vi "Get Write Map.vi"(1 "Setup":T2) -> (0 "Write Map OUT":T1)   [LabVIEW 2024, in "EtherCAT Model.lvlib"]
uses:
  EtherCAT Model.lvlib
  EtherCAT Configuration.ctl
  Write Context Typedef.ctl
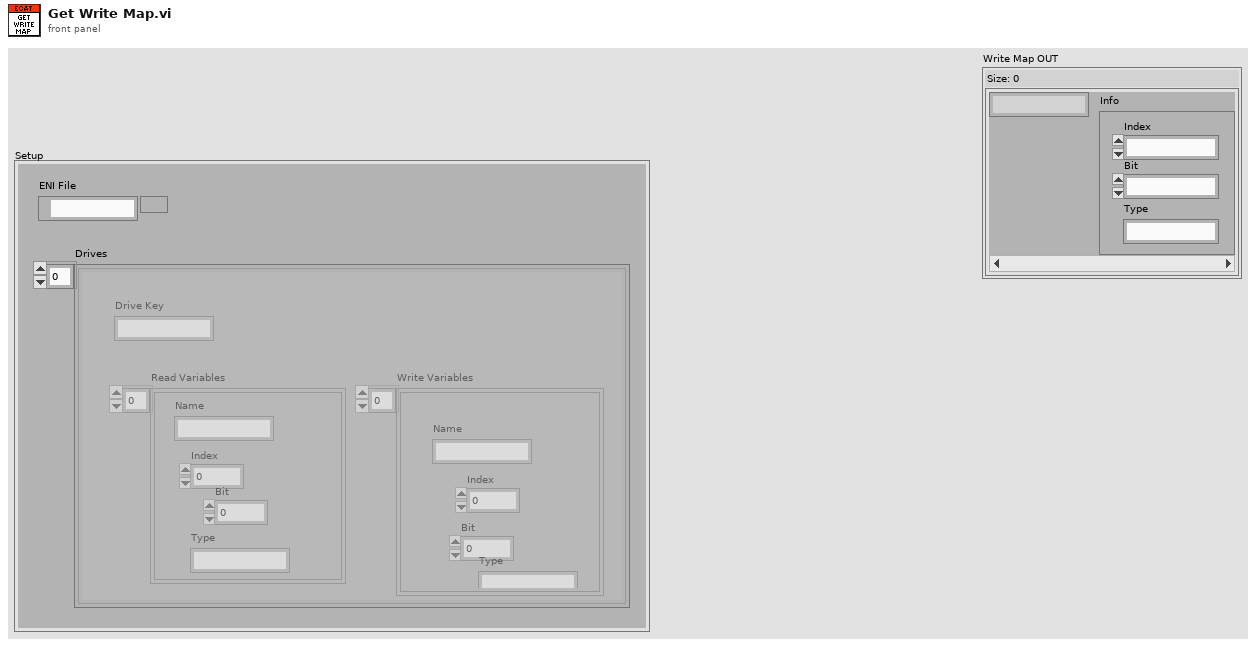
[diagram p1: front panel]
types:
  T1 = typedef "EtherCAT Model.lvlib/Write Context Typedef.ctl" = map{string, cluster{"Index":i32, "Bit":u8, "Type":string}}
  T2 = typedef "EtherCAT Configuration.ctl" = cluster{"ENI File":path, "Drives":cluster{"Drive Key":string, "Read Variables":cluster{"Name":string, "Index":i32, "Bit":u8, "Type":string}[], "Write Variables":cluster{"Name":string, "Index":i32, "Bit":u8, "Type":string}[]}[]}
  T3 = cluster{"Drive Key":string, "Read Variables":cluster{"Name":string, "Index":i32, "Bit":u8, "Type":string}[], "Write Variables":cluster{"Name":string, "Index":i32, "Bit":u8, "Type":string}[]}[]
  T4 = cluster{"Name":string, "Index":i32, "Bit":u8, "Type":string}[]
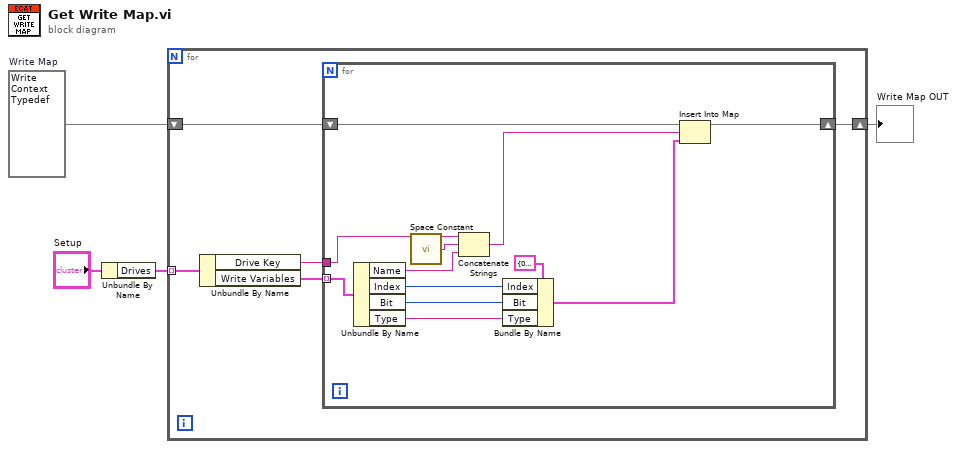
[diagram p0: block diagram]
diagram:
  w2 = T1 {}  # Write Map
  n1 = Unbundle By Name("Setup") -> ("Drives"=w3:T3)
  n2 = for {
    tunnel: w3 -> [w9] mode=indexing
    shift-right: [w5] -> w1
    shift-left: w2 -> [w6]
    n3 = Unbundle By Name(w9) -> ("Drive Key"=w7:string, "Write Variables"=w8:T4)
    n4 = for {
      tunnel: w8 -> [w21] mode=indexing
      tunnel: w7 -> [w20]
      shift-right: [w10] -> w5
      shift-left: w6 -> [w16]
      n5 = Unbundle By Name(w21) -> ("Name"=w18:string, "Index"=w14:i32, "Bit"=w13:u8, "Type"=w12:string)
      n6 = call <vilib>:"Space Constant.vi"() -> ("String"=w19:string)
      n7 = Concatenate Strings(w20, w19, w18) -> (w17:string)
      n8 = Bundle By Name(cluster=cluster{"Index":i32, "Bit":u8, "Type":string} {"Index"=0, "Bit"=0, "Type"=""} ("Info"), "Index"=w14, "Bit"=w13, "Type"=w12) -> (w11:cluster{"Index":i32, "Bit":u8, "Type":string})
      n9 = Insert Into Map(map in=w16, key=w17, value=w11) -> (map out=w10:T1)  [unwired: 2 out]
    }
  }
  "Write Map OUT" <- w1
